vi "Initialise.vi"(6 "View":refnum<vi>, 8 "error in (no error)":errorcluster, 10 "View Buttons":refnum<vi>, 11 "Main Controller Actor in":refnum<class "Main Controller Actor.lvclass">) -> (0 "error out":errorcluster, 3 "Main Controller Actor out":refnum<class "Main Controller Actor.lvclass">, 5 "Observers":cluster{"Actor":refnum<event-registration>})   [LabVIEW 2021, in "Main Controller Actor.lvclass"]
uses:
  Main Controller Actor.lvclass
  C:/dev/LabVIEW/LabMelee/Source/Re-use Libraries/Minimal Actor Framework/Actors/Base Actor/Actor/Actor.lvclass
  Re-use Libraries/Minimal Actor Framework/Messaging/Message/Message.lvclass
  Main Controller Actor.lvclass/Main Controller Actor.ctl
  Re-use Libraries/Minimal Actor Framework/Actors/Base Actor/Actor/Actor.lvclass/Actor.ctl
  Re-use Libraries/Vector 2D/Vector 2D.lvclass
  Launcher/Actor/Glyph.ctl
  Launcher/Actor/Launcher Actor.lvclass
  Error Handler/API/Error Handler Actor API.lvclass
  Launcher/API/Launcher Actor API.lvclass
  <userlib>/_OpenG.lib/file/file.llb/openg_file.lvlib
  Main INI/Main INI.lvlib
  Re-use Libraries/Minimal Actor Framework/Actors/Base Actor/Actor/Actor.lvclass
  Camera/Camera.lvclass
  View.ctl
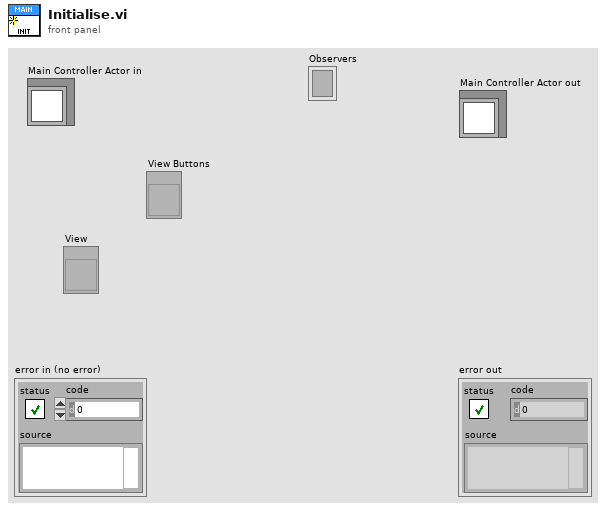
[diagram p1: front panel]
types:
  T1 = typedef "Launcher Actor.lvclass/Glyph.ctl" = u16
  T2 = typedef "Main INI.lvlib/Core Data.ctl" = cluster{"Config":cluster{"System Config Name":string, "Debug":bool}}
  T3 = typedef "Constants.ctl" = cluster{"Colours":cluster{"OK":u32, "Warning":u32, "Error":u32, "Red":u32, "Green":u32, "Blue":u32, "Yellow":u32, "Health":u32, "Energy":u32}, "System":cluster{"Target Frames Second":dbl, "Windows Size":refnum<class "Vector 2D.lvclass">, "World Size":refnum<class "Vector 2D.lvclass">, "Battle Area Size":refnum<class "Vector 2D.lvclass">, "Sidebar Width":sgl, "SC2 Frame Rate [Seconds/Frame]":sgl, "Sidebar Player 2 Y Offset":sgl}, "Game":cluster{"Maximum Asteroids":i32, "Max Energy":i32, "Max Crew":i32, "Maximum Stars":i32}}
  T4 = typedef "Actor.lvclass/Update User Event.ctl" = refnum<user-event>
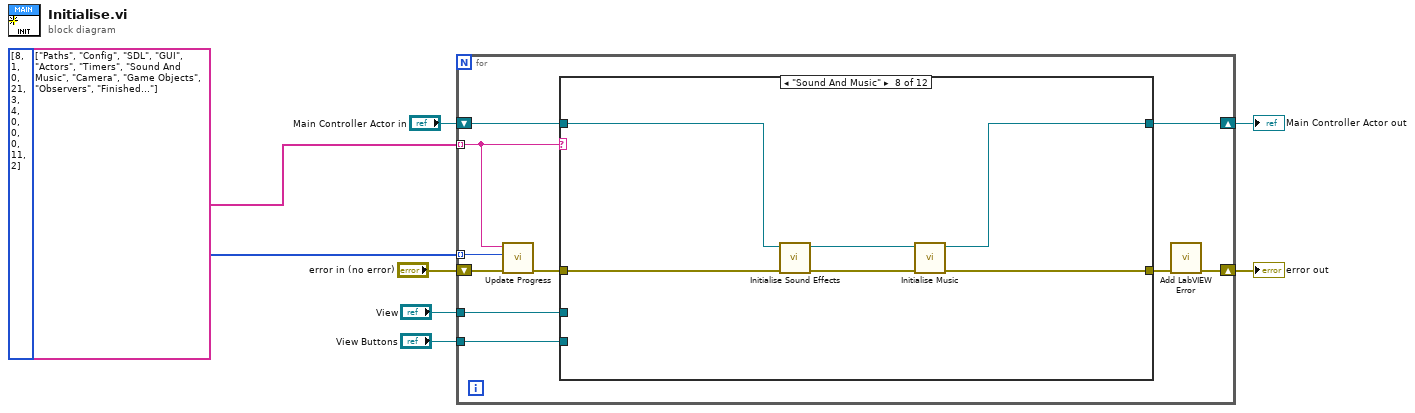
[diagram p0: block diagram]
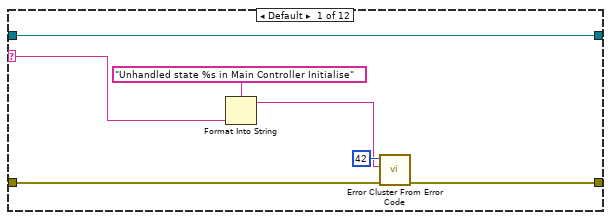
[diagram p2: hidden frame]
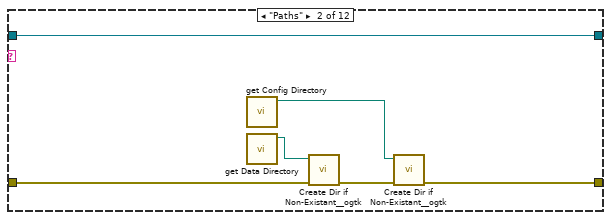
[diagram p3: hidden frame]
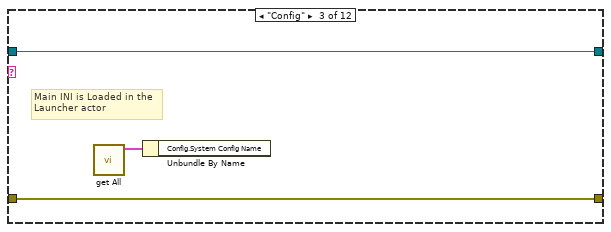
[diagram p4: hidden frame]
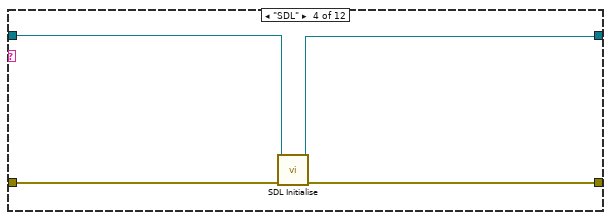
[diagram p5: hidden frame]
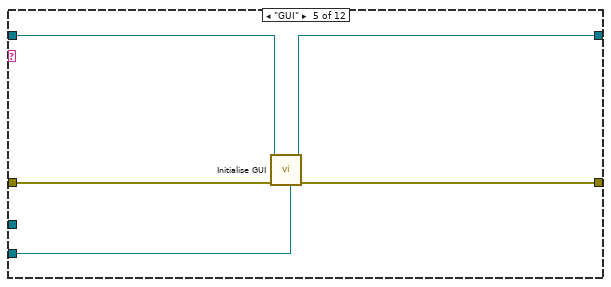
[diagram p6: hidden frame]
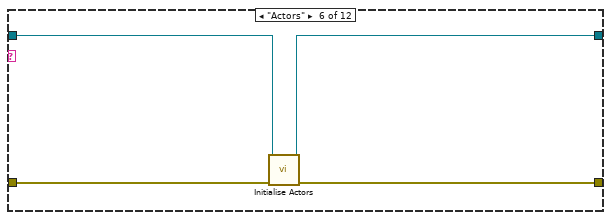
[diagram p7: hidden frame]
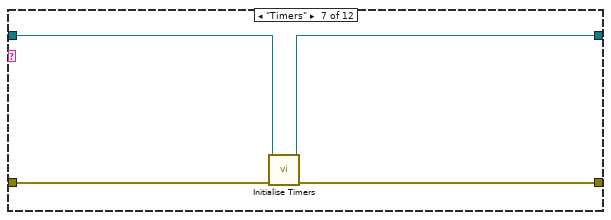
[diagram p8: hidden frame]
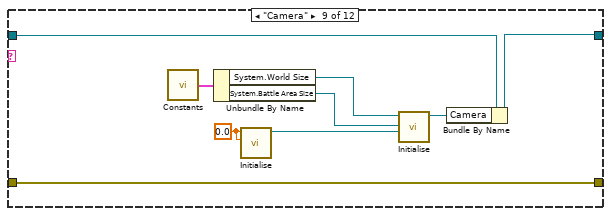
[diagram p9: hidden frame]
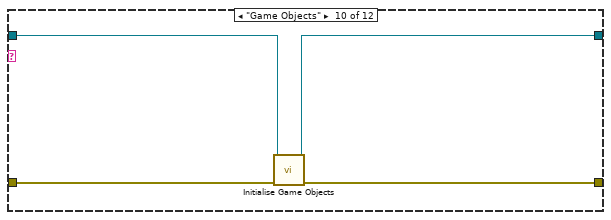
[diagram p10: hidden frame]
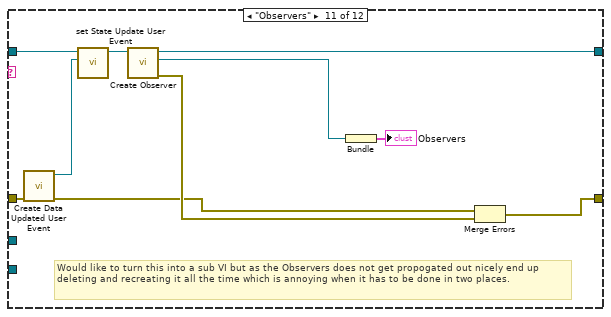
[diagram p11: hidden frame]
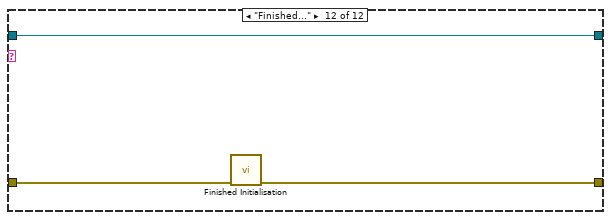
[diagram p12: hidden frame]
diagram:
  n1 = for {
    shift-right: [w16] -> w2
    shift-left: "error in (no error)" -> [w10]
    shift-right: [w14] -> w1
    shift-left: "Main Controller Actor in" -> [w18]
    tunnel: string[] ["Paths", "Config", "SDL", "GUI", "Actors", "Timers", "Sound And Music", "Camera", "Game Objects", "Observers", "Finished..."] -> [w13] mode=indexing
    tunnel: T1[] [8, 1, 0, 21, 3, 4, 0, 0, 0, 11, 2] -> [w12] mode=indexing
    tunnel: "View" -> [w17]
    tunnel: "View Buttons" -> [w9]
    n2 = call "Update Progress.vi"("error in (no error)"=w10, "Glyph"=w12, "Message"=w13) -> ("error out"=w11:errorcluster)  [unwired: 8 in]
    n3 = case shown="\"Sound And Music\"" w13 {
      selector: w13 -> [w20 _ _ _ _ _ _ _ _ _ _ _]
      tunnel: w11 -> [w24 w28 w32 w37 w43 w47 w51 w52 w63 w68 w78 w82]
      tunnel: [w23 w30 w32 w36 w40 w46 w50 w56 w63 w69 w73 w81] -> w15
      tunnel: w18 -> [w25 w29 w33 w38 w42 w45 w49 w54 w66 w67 w79 w83]
      tunnel: [w25 w29 w33 w35 w41 w44 w48 w57 w65 w70 w72 w83] -> w14
      tunnel: w17 -> [_ _ _ _ _ _ _ _ _ _ _ _]
      tunnel: w9 -> [_ _ _ _ w39 _ _ _ _ _ _ _]
      frame Default {
        n4 = Format Into String(format string="Unhandled state %s in Main Controller Initialise", w20) -> (resulting string=w19:string)  [unwired: 2 in, 1 out]
        n5 = call <vilib>:"Error Cluster From Error Code.vi"("error in (no error)"=w24, "error message (\"\")"=w19, "error code (0)"=42) -> ("error out"=w23:errorcluster)  [unwired: 6 in]
      }
      frame "Paths" {
        n6 = call "get Config Directory.vi"() -> ("Config Dir"=w27:path)  [unwired: 11 in]
        n7 = call "get Data Directory.vi"() -> ("Config Dir"=w26:path)  [unwired: 11 in]
        n8 = call <userlib>:"Create Dir if Non-Existant__ogtk.vi"("error in (no error)"=w28, "Directory Path"=w26) -> ("error out"=w31:errorcluster)  [unwired: 7 in, 2 out]
        n9 = call <userlib>:"Create Dir if Non-Existant__ogtk.vi"("error in (no error)"=w31, "Directory Path"=w27) -> ("error out"=w30:errorcluster)  [unwired: 7 in, 2 out]
      }
      frame "Config" {
        # "Main INI is Loaded in the Launcher actor"
        n10 = call "get All.vi"() -> ("Data out"=w34:T2)  [unwired: 10 in, 1 out]
        n11 = Unbundle By Name(w34) -> ()  [unwired: 1 out]
      }
      frame "SDL" {
        n12 = call "SDL Initialise.vi"("error in (no error)"=w37, "Main Controller Actor in"=w38) -> ("error out"=w36:errorcluster, "Main Controller Actor out"=w35:refnum<class "Main Controller Actor.lvclass">)  [unwired: 8 in]
      }
      frame "GUI" {
        n13 = call "Initialise GUI.vi"("View Buttons"=w39, "error in (no error)"=w43, "Main Controller in"=w42) -> ("error out"=w40:errorcluster, "Main Controller out"=w41:refnum<class "Main Controller Actor.lvclass">)  [unwired: 7 in]
      }
      frame "Actors" {
        n14 = call "Initialise Actors.vi"("error in (no error)"=w47, "Main Controller in"=w45) -> ("error out"=w46:errorcluster, "Main Controller out"=w44:refnum<class "Main Controller Actor.lvclass">)  [unwired: 8 in]
      }
      frame "Timers" {
        n15 = call "Initialise Timers.vi"("error in (no error)"=w51, "Main Controller in"=w49) -> ("error out"=w50:errorcluster, "Main Controller out"=w48:refnum<class "Main Controller Actor.lvclass">)  [unwired: 8 in]
      }
      frame "Sound And Music" {
        n16 = call "Initialise Sound Effects.vi"("error in (no error)"=w52, "Main Controller Actor in"=w54) -> ("error out"=w53:errorcluster, "Main Controller Actor out"=w55:refnum<class "Main Controller Actor.lvclass">)  [unwired: 8 in]
        n17 = call "Initialise Music.vi"("error in (no error)"=w53, "Main Controller Actor in"=w55) -> ("error out"=w56:errorcluster, "Main Controller Actor out"=w57:refnum<class "Main Controller Actor.lvclass">)  [unwired: 8 in]
      }
      frame "Camera" {
        w60 = sgl 0.0 ("x")
        n18 = call "Constants.vi"() -> ("Constants"=w62:T3)
        n19 = Unbundle By Name(w62) -> ("System.World Size"=w59:refnum<class "Vector 2D.lvclass">, "System.Battle Area Size"=w58:refnum<class "Vector 2D.lvclass">)
        n20 = call "Initialise.vi"("y"=w60, "x"=w60) -> ("Vector 2D out"=w61:refnum<class "Vector 2D.lvclass">)  [unwired: 9 in]
        n21 = call "Initialise.vi"("Origin"=w61, "View Size"=w58, "World Size"=w59) -> ("Camera out"=w64:refnum<class "Camera.lvclass">)  [unwired: 8 in]
        n22 = Bundle By Name(cluster=w66, "Camera"=w64) -> (w65:refnum<class "Main Controller Actor.lvclass">)
      }
      frame "Game Objects" {
        n23 = call "Initialise Game Objects.vi"("error in (no error)"=w68, "Main Controller Actor in"=w67) -> ("error out"=w69:errorcluster, "Main Controller Actor out"=w70:refnum<class "Main Controller Actor.lvclass">)  [unwired: 8 in]
      }
      frame "Observers" {
        # "Would like to turn this into a sub VI but as the Observers does not get propogated out nicely end up deleting and recreating it all the time which is annoying when it has to be done in two places."
        n24 = call "Create Data Updated User Event.vi"("error in (no error)"=w78) -> ("error out"=w74:errorcluster, "State Update"=w80:T4)  [unwired: 9 in]
        n25 = call "set State Update User Event.vi"("State Update"=w80, "Actor in"=w79) -> ("Actor out"=w77:refnum<class "Main Controller Actor.lvclass">)  [unwired: 9 in]
        n26 = call-dynamic "Create Observer.vi"("Actor in"=w77) -> ("error out"=w75:errorcluster, "Actor"=w76:refnum<event-registration>, "Actor out"=w72:refnum<class "Main Controller Actor.lvclass">)  [unwired: 8 in]
        n27 = Bundle("Actor"=w76) -> (→"Observers":cluster{"Actor":refnum<event-registration>})  [unwired: 1 in]
        n28 = Merge Errors(w74, w75) -> (w73:errorcluster)
      }
      frame "Finished..." {
        n29 = call "Finished Initialisation.vi"("error in (no error)"=w82) -> ("error out"=w81:errorcluster)  [unwired: 10 in]
      }
    }
    n30 = call "Add LabVIEW Error.vi"("error in (no error)"=w15) -> ("error out"=w16:errorcluster)  [unwired: 10 in]
  }
  "error out" <- w2
  "Main Controller Actor out" <- w1
